vi "Release Queue.vi"(8 "error in (no error)":errorcluster, 11 "Messaging in":refnum<class "Messaging.lvclass">) -> (0 "error out":errorcluster, 3 "Messaging out":refnum<class "Messaging.lvclass">)   [LabVIEW 2023, in "Messaging.lvclass"]
uses:
  Messaging.lvclass
  Messaging.lvclass/Messaging.ctl
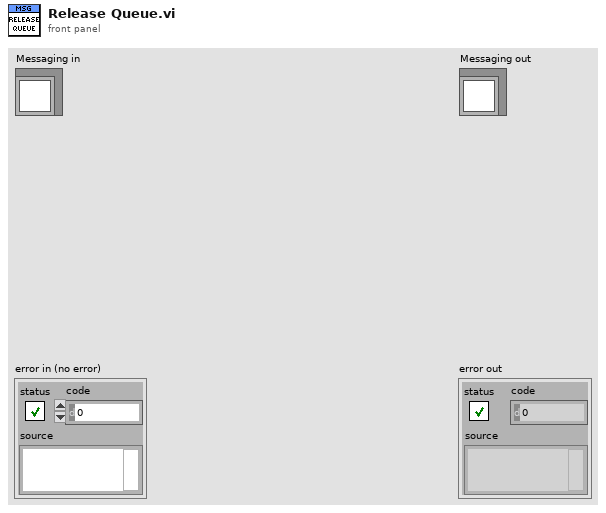
[diagram p1: front panel]
types:
  T1 = typedef "Msg.Q.Ref.ctl" = refnum<queue>
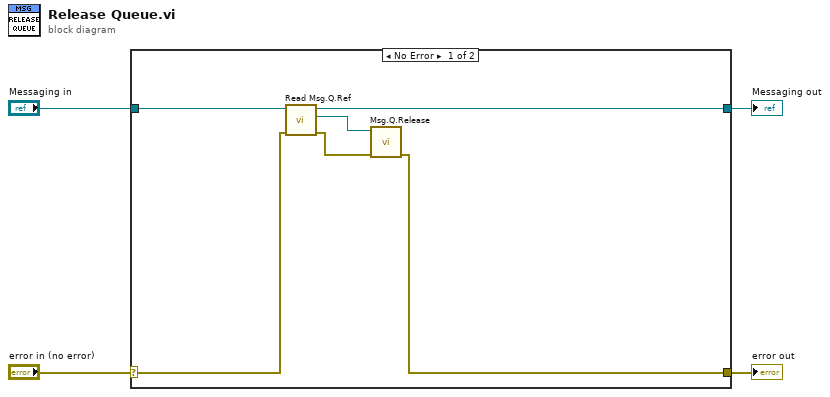
[diagram p0: block diagram]
diagram:
  n1 = case shown="No Error" "error in (no error)" {
    selector: "error in (no error)" -> [w9 w12]
    tunnel: [w6 w12] -> w3
    tunnel: [w5 w11] -> w1
    tunnel: "Messaging in" -> [w10 w11]
    frame No Error {
      n2 = call-dynamic "Read Msg.Q.Ref.vi"("error in (no error)"=w9, "Messaging in"=w10) -> ("error out"=w7:errorcluster, "Msg.Q.Ref"=w8:T1, "Messaging out"=w5:refnum<class "Messaging.lvclass">)  [unwired: 7 in]
      n3 = call "Msg.Q.Release.vi"("Error (in)"=w7, "Msg.Q.Ref"=w8) -> ("Error (out)"=w6:errorcluster)  [unwired: 9 in]
    }
    frame Error {
    }
  }
  "error out" <- w3
  "Messaging out" <- w1
